vi "Create_Object.vi"(8 "error in (no error)":errorcluster, 9 "Block Diagram in":T1, 10 "owner refnum":variant, 11 "Array Control in":refnum<class "Array Control.lvclass">) -> (0 "error out":errorcluster, 1 "Block Diagram Out":T1, 3 "Array Control out":refnum<class "Array Control.lvclass">)   [LabVIEW 2025, in "Array Control.lvclass"]
uses:
  Array Control.lvclass
  C:/Users/mrjak/Documents/GitHub/LVGPT/LabVIEW/VIs/Classes/Node/Node.lvclass
  Controls/bd.ctl
  Node.lvclass
  Controls/wire.ctl
  Controls/Terminal.ctl
  Node.lvclass/Node.ctl
  Array.lvclass
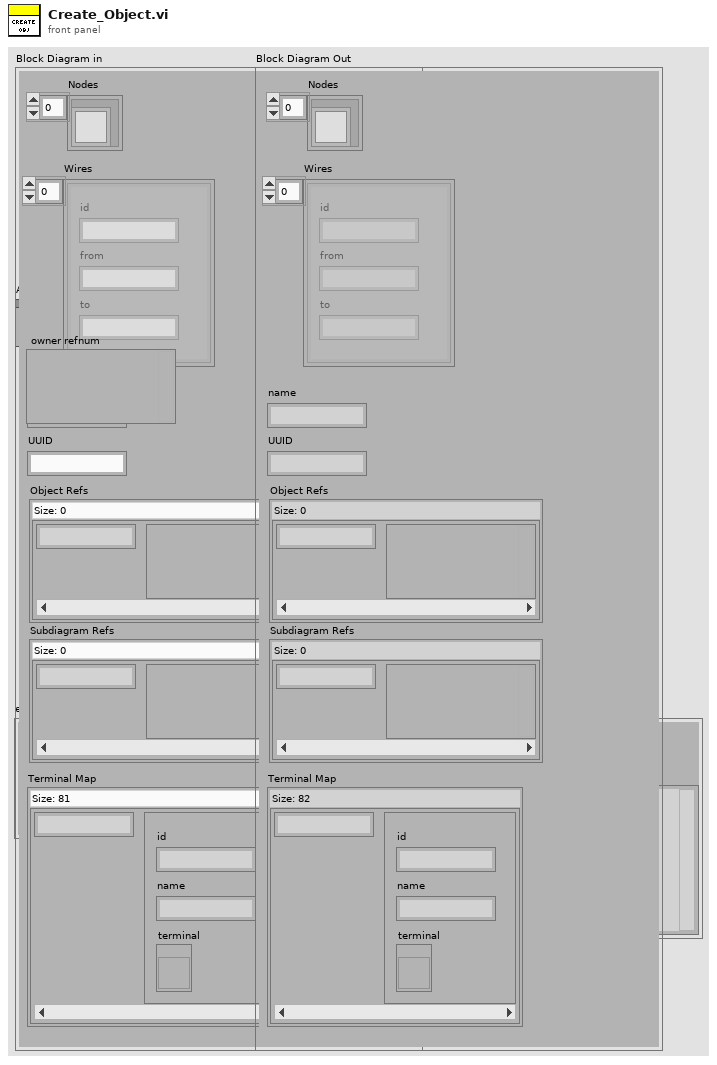
[diagram p1: front panel]
types:
  T1 = typedef "bd.ctl" = cluster{"Nodes":refnum<class "Node.lvclass">[], "Wires":T2[], "name":string, "UUID":string, "Object Refs":map{string, variant}, "Subdiagram Refs":map{string, variant}, "Terminal Map":map{string, T3}}
  T2 = typedef "wire.ctl" = cluster{"id":string, "from":string, "to":string}
  T3 = typedef "Terminal.ctl" = cluster{"id":string, "name":string, "terminal":refnum<vi>}
  T4 = typedef "LVPointTypeDef.ctl" = cluster{"Horizontal":i16, "Vertical":i16}
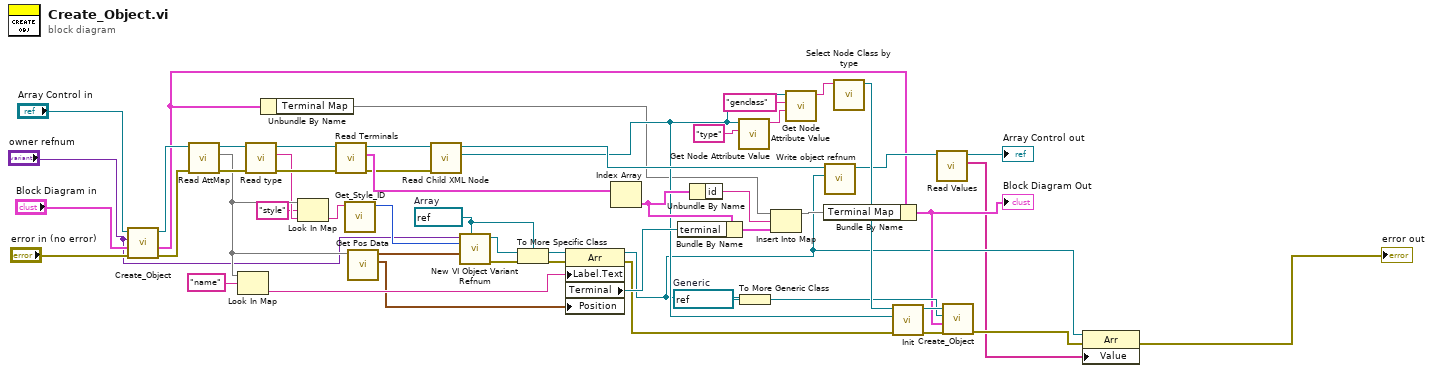
[diagram p0: block diagram]
diagram:
  w16 = refnum<vi> refnum  # Generic
  w12 = refnum<vi> refnum  # Array
  n1 = call-parent "Create_Object.vi"("error in (no error)"="error in (no error)", "Block Diagram in"="Block Diagram in", "owner refnum"="owner refnum", "Node in"="Array Control in") -> ("error out"=w49:errorcluster, "Block Diagram Out"=w9:T1, "Node out"=w48:refnum<class "Array Control.lvclass">)  [unwired: 5 in]
  n2 = call "Read AttMap.vi"("error in (no error)"=w49, "Node in"=w48) -> ("error out"=w46:errorcluster, "AttMap"=w26:map{string, string}, "Node out"=w45:refnum<class "Array Control.lvclass">)  [unwired: 7 in]
  n3 = Look In Map(map=w26, key="name") -> (value=w38:string)  [unwired: 1 in, 1 out]
  n4 = call "Read type.vi"("error in (no error)"=w46, "Node in"=w45) -> ("error out"=w43:errorcluster, "type"=w25:string, "Node out"=w42:refnum<class "Array Control.lvclass">)  [unwired: 7 in]
  n5 = Unbundle By Name(w9) -> ("Terminal Map"=w10:map{string, T3})
  n6 = Look In Map(map=w26, key="style", default value=w25) -> (value=w23:string)  [unwired: 1 out]
  n7 = call "Read Terminals.vi"("error in (no error)"=w43, "Node in"=w42) -> ("error out"=w32:errorcluster, "Terminals"=w33:T3[], "Node out"=w31:refnum<class "Array Control.lvclass">)  [unwired: 7 in]
  n8 = call "Get_Style_ID.vi"("Style"=w23) -> ("style"=w44:i32)  [unwired: 8 in, 2 out]
  n9 = call "Get Pos Data.vi"("AttMap"=w26) -> ("FP Position"=w6:T4, "Position"=w47:T4)  [unwired: 9 in]
  n10 = call-dynamic "Read Child XML Node.vi"("error in (no error)"=w32, "Array in"=w31) -> ("Child XML Node"=w19:refnum<k20>, "Array out"=w27:refnum<class "Array Control.lvclass">)  [unwired: 7 in, 1 out]
  n11 = call "New VI Object Variant Refnum.vi"("vi object class"=w12, "location"=w47, "style"=w44, "owner refnum"="owner refnum") -> ("error out"=w39:errorcluster, "object refnum"=w40:refnum<vi>)  [unwired: 6 in]
  n12 = To More Specific Class(target class=w12, reference=w40) -> (specific class reference=w13:refnum<vi>)  [unwired: 1 in, 1 out]
  n13 = property class="Arr"(reference=w13, error in=w39, "Label.Text"=w38, "Position"=w6) -> (reference out=w3:refnum<vi>, error out=w20:errorcluster, "Terminal"=w34:refnum<vi>)
  n14 = Index Array(array=w33) -> (element=w36:T3)  [unwired: 1 in]
  n15 = Bundle By Name(cluster=w36, "terminal"=w34) -> (w35:T3)
  n16 = Unbundle By Name(w36) -> ("id"=w37:string)
  n17 = call "Get Node Attribute Value.vi"("Attribute Name"="type", "Refnum in"=w19) -> ("Value"=w29:string)  [unwired: 9 in]
  n18 = To More Generic Class(target class=w16, reference=w3) -> (generic class reference=w14:refnum<vi>)
  n19 = Insert Into Map(map in=w10, key=w37, value=w35) -> (map out=w8:map{string, T3})  [unwired: 2 out]
  n20 = call "Get Node Attribute Value.vi"("Default Value"=w29, "Attribute Name"="genclass", "Refnum in"=w19) -> ("Value"=w22:string)  [unwired: 8 in]
  n21 = Bundle By Name(cluster=w9, "Terminal Map"=w8) -> (w7:T1)
  "Block Diagram Out" <- w7
  n22 = call-dynamic "Write object refnum.vi"("object refnum"=w3, "Node in"=w27) -> ("Node out"=w11:refnum<class "Array Control.lvclass">)  [unwired: 8 in, 1 out]
  n23 = call "Select Node Class by type.vi"("Value"=w22) -> ("Node out"=w21:refnum<class "Node.lvclass">)  [unwired: 10 in]
  n24 = call-dynamic "Init.vi"("error in (no error)"=w20, "Node Reg"=w19, "Node in"=w21) -> ("error out"=w18:errorcluster, "Node out"=w17:refnum<class "Node.lvclass">)  [unwired: 7 in]
  n25 = call-dynamic "Read Values.vi"("Array in"=w11) -> ("Values"=w2:string[], "Array out"=→"Array Control out":refnum<class "Array Control.lvclass">)  [unwired: 8 in, 1 out]
  n26 = call-dynamic "Create_Object.vi"("error in (no error)"=w18, "Block Diagram in"=w7, "owner refnum"=w14, "Node in"=w17) -> ("error out"=w4:errorcluster)  [unwired: 5 in, 2 out]
  n27 = property class="Arr"(reference=w3, error in=w4, "Value"=w2) -> (error out=→"error out":errorcluster)  [unwired: 1 out]
